vi "Destroy to Listener.vi"(8 "Error In":errorcluster, 10 "Channel":refnum<class "Channel.lvclass">, 11 "Listener In":refnum<class "Listener.lvclass">) -> (0 "Error Out":errorcluster, 3 "Listener Out":refnum<class "Listener.lvclass">)   [LabVIEW 2018, in "Toolkit.lvlib" / "Channel.lvclass"]
doc: "Passes through the Listener and destroys this Channel object."
uses:
  Channel.lvclass
  Listener/Listener.lvclass
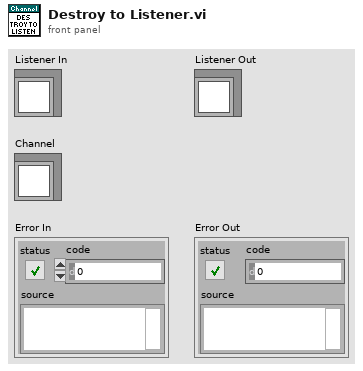
[diagram p1: front panel]
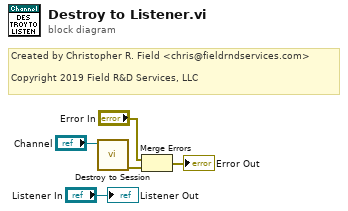
[diagram p0: block diagram]
diagram:
  # "Created by Christopher R. Field <chris@fieldrndservices.com>\n\nCopyright 2019 Field R&D Services, LLC"
  n1 = call "Destroy to Session.vi"("Channel"="Channel") -> ("Error Out"=w1:errorcluster)  [unwired: 9 in, 1 out]
  n2 = Merge Errors("Error In", w1) -> (→"Error Out":errorcluster)
  "Listener Out" <- "Listener In"
